vi "Overlay LineOut XDisplay.vi"(7 "Group":string, 8 "error in":errorcluster, 9 "LineCoord":i32[](array[numeric]), 10 "Calibration":dbl=1.0, 11 "Image In":T1) -> (0 "error out":errorcluster, 1 "Image Out":T1, 2 "FWHM":dbl, 3 "Line Graph":cluster{"x0":sgl, "dx":sgl, "Pixels Line":sgl[]})   [LabVIEW 2009, in "POLARIS IMAQ Display.xctl"]
doc: "creates overlay poligon line for a trend. If slope of the line is les 45° trend appears at bottom border otherwise at the left border. \n\nthanks for idee and first implementation to Sebastian Keppler, FSU-IOQ\n\nauthor: Alexander Kessler, Helmholtz-Institut-Jena \nmaintainer: Alexander Kessler: alexander.kessler@uni-jena.de\n\n\n\nLicense Agreement for this software:\n\nCopyright (C)\nHelmholtz-Institut-Jena\nFröbelstieg 3\n07743 Jena\nGermany\n\nThis program is free software; you can redistribute it and/or modify it under the terms of the GNU General Public License as published by the Free Software Foundation; either version 2 of the license, or (at your option) any later version.\n\nThis program is distributed in the hope that it will be useful, but WITHOUT ANY WARRANTY; without even the implied warranty of MERCHANTABILITY or FITNESS FOR A PARTICULAR PURPOSE. See the GNU General License for more details (http://www.gnu.org)."
uses:
  POLARIS IMAQ Display.xctl
  <vilib>/vision/Image Controls.llb/IMAQ Image.ctl
  <vilib>/vision/NI_Vision_Development_Module.lvlib
  <vilib>/Analysis/NI_AALBase.lvlib
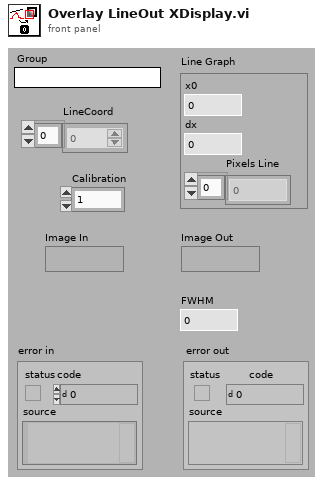
[diagram p1: front panel]
types:
  T1 = typedef "IMAQ Image.ctl" = refnum<image>
  T2 = cluster{"Min":sgl, "Max":sgl, "Mean":sgl, "Std Dev":sgl, "Count":i32}
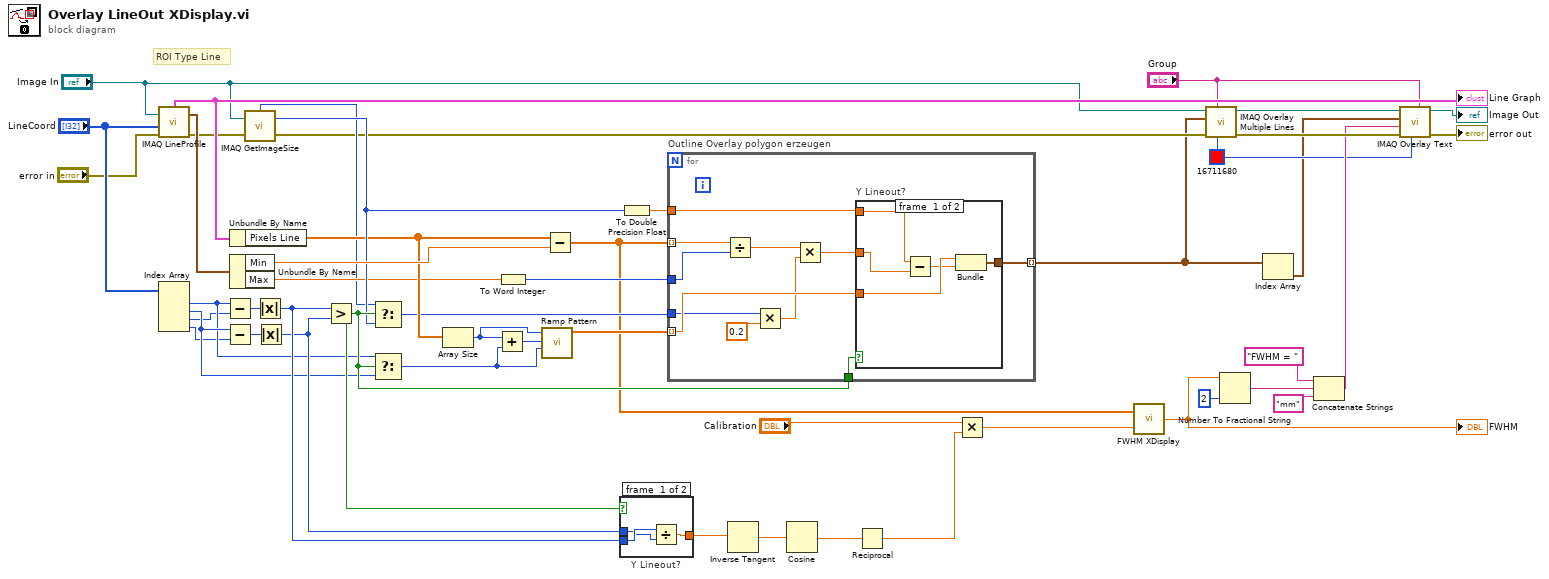
[diagram p0: block diagram]
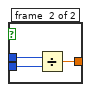
[diagram p2: hidden frame]
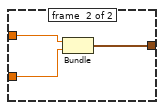
[diagram p3: hidden frame]
diagram:
  w8 = u32 16711680 ("Color")
  # "ROI Type Line"
  n1 = call "IMAQ LineProfile"("error in (no error)"="error in", "Line Coordinates"="LineCoord", "Image"="Image In") -> ("error out"=w23:errorcluster, "Line Graph"=w36:cluster{"x0":sgl, "dx":sgl, "Pixels Line":sgl[]}, "Line Information"=w33:T2)  [unwired: 2 in, 1 out]
  "Line Graph" <- w36
  n2 = Index Array(array="LineCoord") -> (element #1=w41:i32, element #2=w42:i32, element #3=w32:i32, element #4=w27:i32)  [unwired: 4 in]
  n3 = Subtract(x=w41, y=w32) -> (x-y=w28:i32)
  n4 = Subtract(x=w42, y=w27) -> (x-y=w29:i32)
  n5 = Unbundle By Name(w36) -> ("Pixels Line"=w37:sgl[])
  n6 = Unbundle By Name(w33) -> ("Min"=w45:sgl, "Max"=w34:sgl)
  n7 = call "IMAQ GetImageSize"("Image"="Image In", "error in (no error)"=w23) -> ("Y Resolution"=w43:i32, "X Resolution"=w30:i32, "error out"=w24:errorcluster)  [unwired: 2 in]
  n8 = Absolute Value(x=w28) -> (abs(x)=w48:i32)
  n9 = Absolute Value(x=w29) -> (abs(x)=w47:i32)
  n10 = Greater?(x=w48, y=w47) -> (0:w46:bool)
  n11 = Select(t=w30, s=w46, f=w43) -> (s? t:f=w31:i32)
  n12 = Select(t=w41, s=w46, f=w42) -> (s? t:f=w39:i32)
  n13 = Array Size(array=w37) -> (size(s)=w38:i32)
  n14 = Add(x=w38, y=w39) -> (x+y=w40:i32)
  n15 = To Word Integer(number=w34) -> (16bit integer=w35:i16)
  n16 = call <vilib>:"Ramp Pattern.vi"("start"=w39, "end"=w40, "samples"=w38) -> ("Ramp Pattern"=w20:dbl[])  [unwired: 7 in, 1 out]
  n17 = Subtract(x=w37, y=w45) -> (x-y=w7:sgl[])
  n18 = case "Y Lineout?" shown="True" w46 {
    tunnel: w47 -> [w51 w55]
    tunnel: w48 -> [w52 w54]
    tunnel: [w50 w53] -> w11
    frame #0 {
      n19 = Divide(x=w52, y=w51) -> (x/y=w50:dbl)
    }
    frame #1 {
      n20 = Divide(x=w55, y=w54) -> (x/y=w53:dbl)
    }
  }
  n21 = To Double Precision Float(number=w43) -> (double precision float=w44:dbl)
  n22 = for "Outline Overlay polygon erzeugen" {
    tunnel: w20 -> [w64] mode=indexing
    tunnel: w7 -> [w63] mode=indexing
    tunnel: [w66] -> w3 mode=indexing
    tunnel: w35 -> [w61]
    tunnel: w31 -> [w59]
    tunnel: w46 -> [w57]
    tunnel: w44 -> [w56]
    n23 = Divide(x=w63, y=w61) -> (x/y=w62:sgl)
    n24 = Multiply(x=w59, y=0.2) -> (x*y=w58:dbl)
    n25 = Multiply(x=w62, y=w58) -> (x*y=w65:dbl)
    n26 = case "Y Lineout?" shown="False" w57 {
      tunnel: [w71 w74] -> w66
      tunnel: w65 -> [w69 w73]
      tunnel: w64 -> [w70 w72]
      tunnel: w56 -> [w67 _]
      frame #0 {
        n27 = Subtract(x=w67, y=w69) -> (x-y=w68:dbl)
        n28 = Bundle(w70, w68) -> (w71:cluster{dbl, dbl})  [unwired: 1 in]
      }
      frame #1 {
        n29 = Bundle(w73, w72) -> (w74:cluster{dbl, dbl})  [unwired: 1 in]
      }
    }
  }
  n30 = Inverse Tangent(1:w11) -> (0:w12:dbl)
  n31 = Cosine(x=w12) -> (cos(x)=w10:dbl)
  n32 = Reciprocal(x=w10) -> (1/x=w9:dbl)
  n33 = Multiply(x="Calibration", y=w9) -> (x*y=w6:dbl)
  n34 = call "FWHM XDisplay.vi"("calibration"=w6, "array"=w7) -> ("FHWM"=w5:dbl)
  "FWHM" <- w5
  n35 = call "IMAQ Overlay Multiple Lines"("Color"=w8, "Group"="Group", "error in (no error)"=w24, "Line End Points"=w3, "Image"="Image In") -> ("error out"=w25:errorcluster, "Image Out"=w21:T1)  [unwired: 5 in]
  n36 = Number To Fractional String(number=w5, precision (6)=i16 2) -> (F-format string=w17:string)  [unwired: 2 in]
  n37 = Index Array(array=w3) -> (element=w2:cluster{dbl, dbl})  [unwired: 1 in]
  n38 = Concatenate Strings("FWHM = " ("string"), w17, "mm" ("string")) -> (w14:string)
  n39 = call "IMAQ Overlay Text"("Group"="Group", "Text Color (black)"=w8, "error in (no error)"=w25, "String"=w14, "Origin"=w2, "Image"=w21) -> ("error out"=→"error out":errorcluster, "Image Out"=→"Image Out":T1)  [unwired: 4 in]
